vi "DetectTrajectoryCollision.vi"(4 "ball":dbl[](array[numeric]), 5 "IA State":T1={"our_robots"=[], "enemy_robots"=[], "balls"=[], "geometry"={"line_width"=0, "field_length"=0, "field_width"=0, "boundary_width"=0, "referee_width"=0, "goal_width"=0, "goal_depth"=0, "goal_wall_width"=0, "center_circle_radius"=0, "defense_radius"=0, "defense_stretch"=0, "free_kick_from_defense_dist"=0, "penalty_spot_from_field_line_dist"=0, "penalty_line_from_spot_dist"=0}, "IA Judge"={"stage"="", "command"="", "our_goalie_id"=0.0, "enemy_goalie_id"=0.0, "command enum"=enum."Halt", "Time"=enum."Azul"}, "Received Timestamp"=timestamp(0 s since 1904-01-01), "Events"={"Touch"=FALSE, "Ball out"=FALSE, "id touch"=0.0, "Ball out of \nVision"=FALSE, "Ball inside \nGoalie area"=FALSE, "Robot not responding"=FALSE, "Robots responding status"=[1.0, 1.0, 1.0, 1.0, 1.0, 1.0], "Enemy Ball \nPossession"=FALSE, "Pass State"=FALSE, "id end of pass"=0.0, "Kick"=FALSE, "Id ini Possession"=0.0, "Ball Possesion"=FALSE, "Id Possesion"=0.0, "Direct Kick"=FALSE, "2nd Strk Ativo"=FALSE}}, 6 "our_robots":T2[](array[typedef]), 7 "Robot in":T2={"id"=0, "function"=enum."Attacker", "x"=0.0, "y"=0.0, "orientation"=0.0, "v_tangent"=0.0, "v_normal"=0.0, "v_ang"=0.0, "kick_x"=0.0, "kick_z"=0.0, "dribble"=FALSE, "Timestamp"=timestamp(0 s since 1904-01-01), "estimatives"={"est_v_tangent"=0.0, "est_v_normal"=0.0, "est_vx"=0.0, "est_vy"=0.0, "Pos Robot Est"=[]}, "dest_x_kick"=0.0, "dest_y_kick"=0.0, "Gap Coord"=[], "States"=enum."Pass", "Path "=[], "Path  Smooth"=[], "Dest"=[]}, 8 "Goal":dbl[](array[numeric]), 9 "Initial State":dbl[](array[numeric]), 10 "Last Path":dbl[][](array[numeric]), 11 "enemy_robots":T2[](array[typedef])) -> (2 "Collision":bool)   [LabVIEW 2018]
uses:
  Core/AI Robot.ctl
  Intel/Functions Enum.ctl
  Intel/AttackerStates.ctl
  PathDests.ctl
  PathDest.ctl
  Core/AI Input.ctl
  Core/AI Ball.ctl
  Core/Field Size.ctl
  Core/AI Judge.ctl
  Intel/Command Enum.ctl
  Util/Events/Events.ctl
  <vilib>/Analysis/NI_AALPro.lvlib
  <vilib>/Analysis/_algsub.llb/Real Vector Norm.vi
panel:
  out "Is there colision?":bool
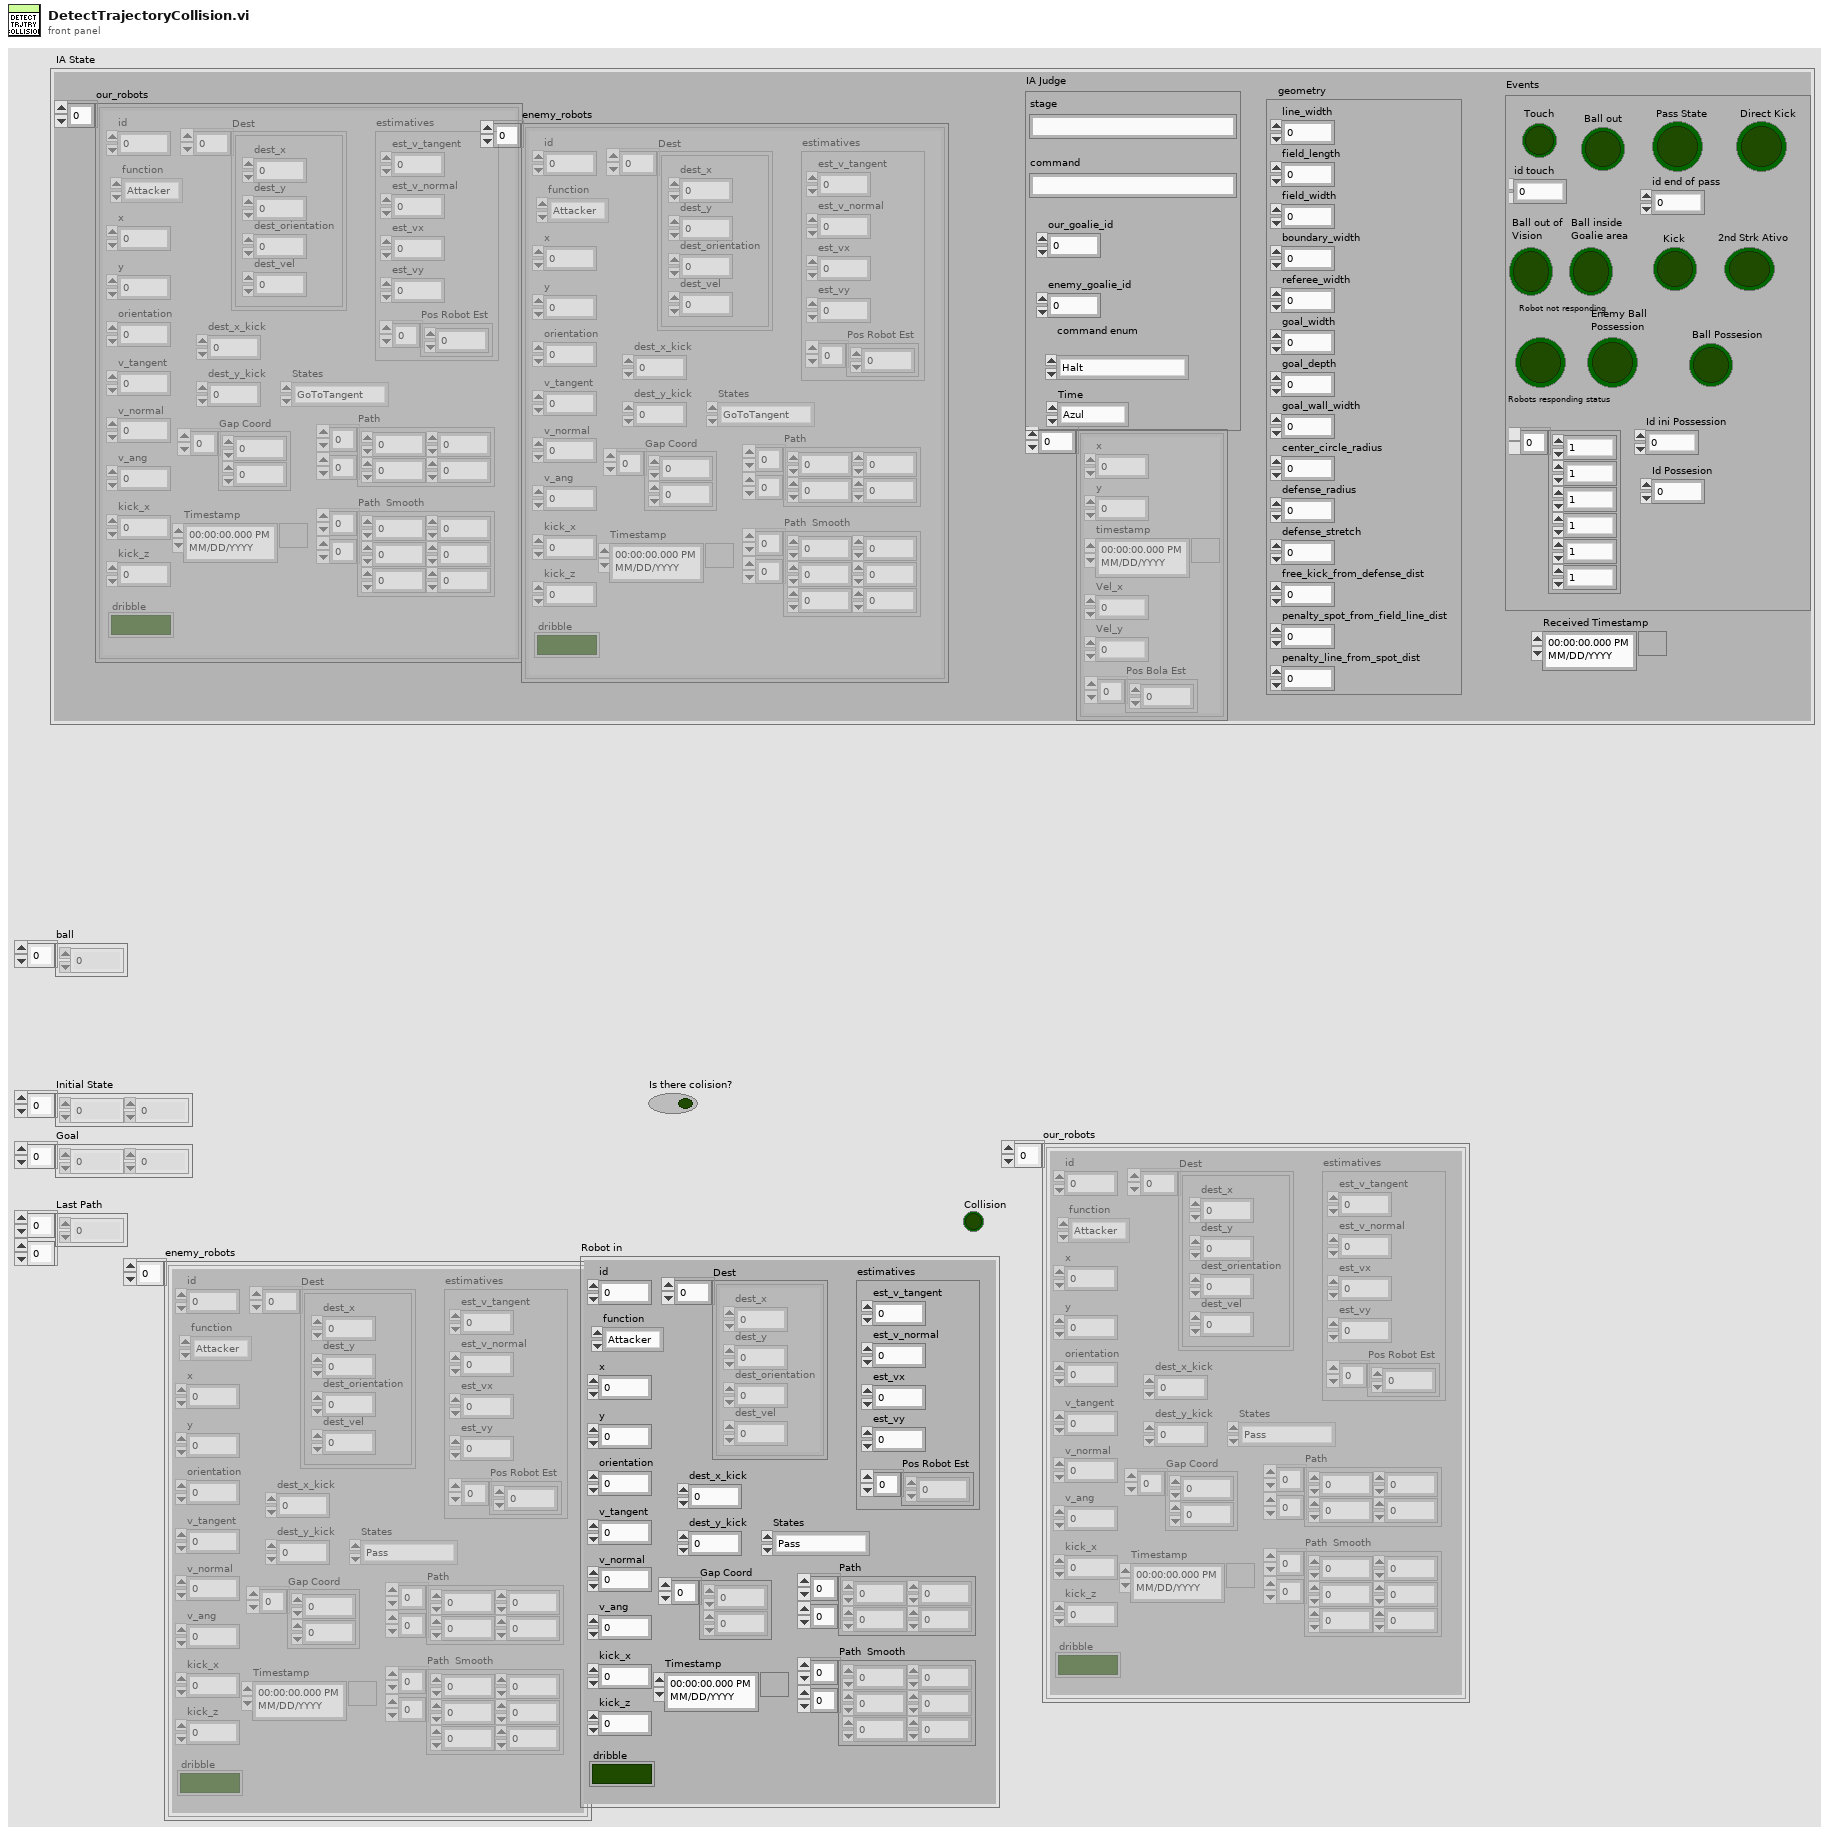
[diagram p1: front panel]
types:
  T1 = typedef "AI Input.ctl" = cluster{"our_robots":T2[], "enemy_robots":T2[], "balls":T7[], "geometry":T8, "IA Judge":T9, "Received Timestamp":timestamp, "Events":T11}
  T2 = typedef "AI Robot.ctl" = cluster{"id":u32, "function":T3, "x":dbl, "y":dbl, "orientation":dbl, "v_tangent":dbl, "v_normal":dbl, "v_ang":dbl, "kick_x":dbl, "kick_z":dbl, "dribble":bool, "Timestamp":timestamp, "estimatives":cluster{"est_v_tangent":dbl, "est_v_normal":dbl, "est_vx":dbl, "est_vy":dbl, "Pos Robot Est":dbl[]}, "dest_x_kick":dbl, "dest_y_kick":dbl, "Gap Coord":dbl[], "States":T4, "Path ":dbl[][], "Path  Smooth":dbl[][], "Dest":T5}
  T3 = typedef "Functions Enum.ctl" = enum16{"2nd Striker", "Attacker", "Goalie", "Defender", "Striker", "Goto 0", "Dummy", "Kicker", "ZigZag 0", "ZigZag 1", "ZigZag 2", "ZigZag 3", "ZigZag 4", "ZigZag 5", "ZigZag 6", "ZigZag 7", "ZigZag 8", ""}
  T4 = typedef "AttackerStates.ctl" = enum16{"Pass", "GoToTangent", "BallGetting", "GoToKick", ""}
  T5 = typedef "PathDests.ctl" = T6[]
  T6 = typedef "PathDest.ctl" = cluster{"dest_x":dbl, "dest_y":dbl, "dest_orientation":dbl, "dest_vel":dbl}
  T7 = typedef "AI Ball.ctl" = cluster{"x":dbl, "y":dbl, "timestamp":timestamp, "Vel_x":dbl, "Vel_y":dbl, "Pos Bola Est":dbl[]}
  T8 = typedef "Field Size.ctl" = cluster{"line_width":u32, "field_length":u32, "field_width":u32, "boundary_width":u32, "referee_width":u32, "goal_width":u32, "goal_depth":u32, "goal_wall_width":u32, "center_circle_radius":u32, "defense_radius":u32, "defense_stretch":u32, "free_kick_from_defense_dist":u32, "penalty_spot_from_field_line_dist":u32, "penalty_line_from_spot_dist":u32}
  T9 = typedef "AI Judge.ctl" = cluster{"stage":string, "command":string, "our_goalie_id":dbl, "enemy_goalie_id":dbl, "command enum":T10, "Time":enum16{"Azul", "Amarelo"}}
  T10 = typedef "Command Enum.ctl" = enum16{"Halt", "Stop", "Force Start", "PKA Normal Start", "Prepare Kickoff Ally", "PKE Normal Start", "Prepare Kickoff Enemy", "Prepare Penalty Ally", "PPA Normal Start", "Prepare Penalty Enemy", "PPE Normal Start", "Direct Free Enemy", "Direct Free Ally", "Indirect Free Enemy", "Indirect Free Ally", "Timeout Enemy", "Timeout Ally", "Goal Enemy", "Goal Ally", "Ball Placement Enemy", "Ball Placement Ally", "Normal Half Time", "Extra Time Break", "Extra Half Time", "None", "Post Game"}
  T11 = typedef "Events.ctl" = cluster{"Touch":bool, "Ball out":bool, "id touch":dbl, "Ball out of \nVision":bool, "Ball inside \nGoalie area":bool, "Robot not responding":bool, "Robots responding status":dbl[], "Enemy Ball \nPossession":bool, "Pass State":bool, "id end of pass":dbl, "Kick":bool, "Id ini Possession":dbl, "Ball Possesion":bool, "Id Possesion":dbl, "Direct Kick":bool, "2nd Strk Ativo":bool}
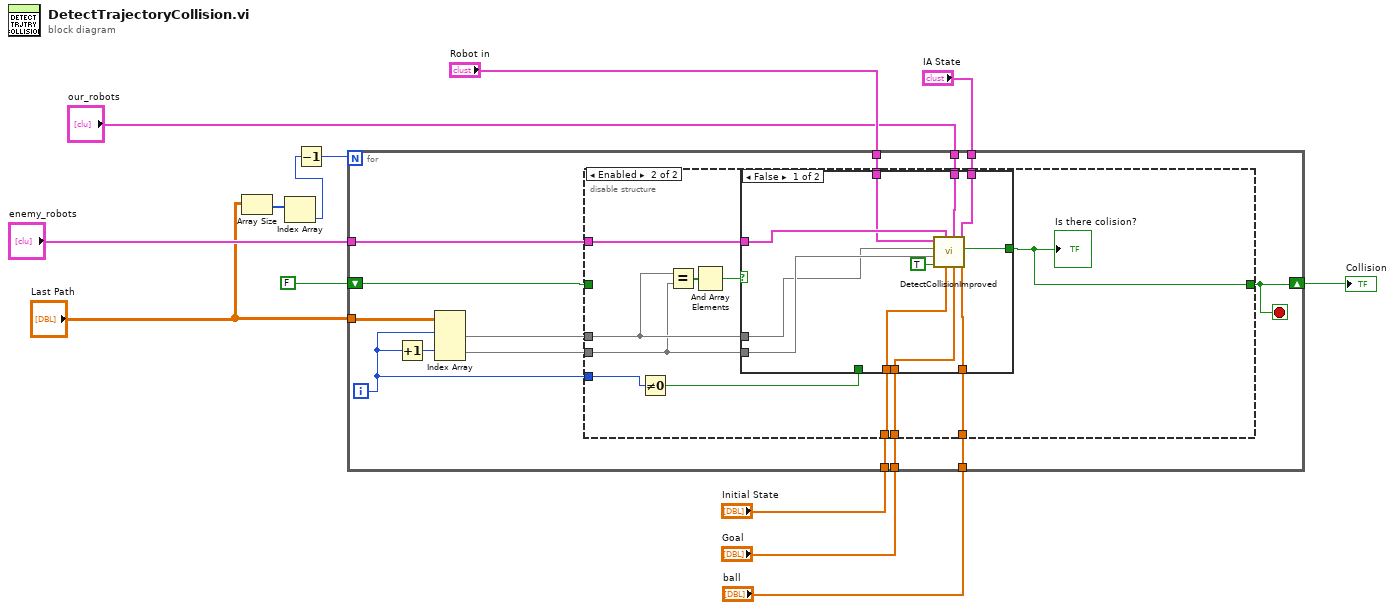
[diagram p0: block diagram]
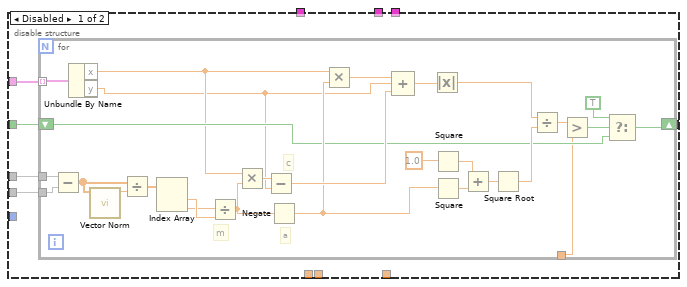
[diagram p2: hidden frame]
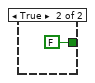
[diagram p3: hidden frame]
diagram:
  n1 = Array Size(array="Last Path") -> (size(s)=w10:i32[])
  n2 = Index Array(array=w10) -> (element=w5:i32)  [unwired: 1 in]
  n3 = Decrement(x=w5) -> (x-1=w6:i32)
  n4 = for {
    N: w6 -> [_]
    tunnel: "enemy_robots" -> [w27]
    tunnel: "Last Path" -> [w26]
    shift-right: [w22] -> w4
    shift-left: FALSE -> [w23]
    tunnel: "Robot in" -> [w19]
    tunnel: "Initial State" -> [w18]
    tunnel: "Goal" -> [w17]
    tunnel: "our_robots" -> [w16]
    tunnel: "ball" -> [w15]
    tunnel: "IA State" -> [w14]
    i -> [w20]
    stop <- w22 stop-if-true
    n5 = Increment(x=w20) -> (x+1=w21:i32)
    n6 = Index Array(array=w26, index (row) #1=w20, index (row) #2=w21) -> (element #1=w25:dbl[], element #2=w24:dbl[])  [unwired: 2 in]
    n7 = disable-structure shown="Enabled" {
      disable-tunnel: w27 -> [w32 w72]
      disable-tunnel: w25 -> [w31 w67]
      disable-tunnel: w24 -> [w30 w66]
      disable-tunnel: w23 -> [w29 _]
      disable-tunnel: [w28 w68] -> w22
      disable-tunnel: w20 -> [_ w74]
      disable-tunnel: w19 -> [_ w73]
      disable-tunnel: w18 -> [_ w70]
      disable-tunnel: w17 -> [_ w69]
      disable-tunnel: w16 -> [_ w63]
      disable-tunnel: w15 -> [_ w62]
      disable-tunnel: w14 -> [_ w61]
      frame Disabled {
        n8 = for {
          tunnel: w32 -> [w53] mode=indexing
          tunnel: w31 -> [w60]
          tunnel: w30 -> [w59]
          tunnel: _ -> [w33]
          shift-right: [w40] -> w28
          shift-left: w29 -> [w38]
          # "c"
          # "a"
          # "m"
          n9 = Subtract(x=w60, y=w59) -> (x-y=w57:dbl[])
          n10 = Unbundle By Name(w53) -> ("x"=w35:dbl, "y"=w34:dbl)
          n11 = call-poly <vilib>:"Vector Norm.vi"("Input Vector"=w57) -> ("norm"=w58:dbl)  [unwired: 9 in, 1 out]
          n12 = Divide(x=w57, y=w58) -> (x/y=w56:dbl[])
          n13 = Index Array(array=w56) -> (element #1=w55:dbl, element #2=w36:dbl)  [unwired: 2 in]
          n14 = Divide(x=w36, y=w55) -> (x/y=w54:dbl)
          n15 = Multiply(x=w35, y=w54) -> (x*y=w37:dbl)
          n16 = Subtract(x=w37, y=w34) -> (x-y=w51:dbl)
          n17 = Negate(x=w54) -> (-x=w47:dbl)
          n18 = Multiply(x=w35, y=w47) -> (x*y=w52:dbl)
          n19 = Compound Arithmetic op=ADD(w52, w34, w51) -> (w50:dbl)
          n20 = Absolute Value(x=w50) -> (abs(x)=w44:dbl)
          n21 = Square(x=1.0) -> (x^2=w49:dbl)
          n22 = Square(x=w47) -> (x^2=w48:dbl)
          n23 = Add(x=w49, y=w48) -> (x+y=w45:dbl)
          n24 = Square Root(x=w45) -> (sqrt(x)=w43:dbl)
          n25 = Divide(x=w44, y=w43) -> (x/y=w42:dbl)
          n26 = Greater?(x=w42, y=w33) -> (0:w41:bool)
          n27 = Select(t=TRUE, s=w41, f=w38) -> (s? t:f=w40:bool)
        }
      }
      frame Enabled {
        n28 = Not Equal To 0?(x=w74) -> (x != 0?=w71:bool)
        n29 = Equal?(x=w67, y=w66) -> (x = y?=w65:bool[])
        n30 = And Array Elements(Boolean array=w65) -> (logical AND=w64:bool)
        n31 = case shown="False" w64 {
          tunnel: w73 -> [w79 _]
          tunnel: w72 -> [w80 _]
          tunnel: w66 -> [w85 _]
          tunnel: w67 -> [w84 _]
          tunnel: w71 -> [_ _]
          tunnel: w70 -> [w83 _]
          tunnel: w69 -> [w78 _]
          tunnel: [w81 FALSE ("Is there colision?")] -> w68
          tunnel: w63 -> [w77 _]
          tunnel: w62 -> [w76 _]
          tunnel: w61 -> [w75 _]
          frame False {
            n32 = call "DetectCollisionImproved.vi"("ball"=w76, "IA State"=w75, "Goal"=w78, "our_robots"=w77, "Initial State"=w83, "enemy_robots"=w80, "Is not first robot?"=TRUE, "element being analyzed"=w85, "element already in path"=w84, "Robot in"=w79) -> ("Is there colision?"=w81:bool)  [unwired: 1 in]
          }
          frame True {
          }
        }
        "Is there colision?" <- w68
      }
    }
  }
  "Collision" <- w4
